vi "Image_set.vi"(8 "error in (no error)":errorcluster, 10 "Image":T1) -> (0 "error out":errorcluster)   [LabVIEW 2009, in "NetworkVarTarget.lvlib"]
uses:
  NetworkVarTarget.lvlib
  <vilib>/vision/Image Controls.llb/IMAQ Image.ctl
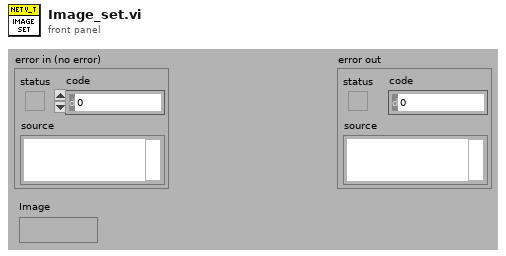
[diagram p1: front panel]
types:
  T1 = typedef "IMAQ Image.ctl" = refnum<image>
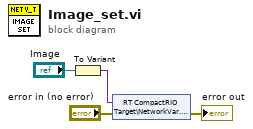
[diagram p0: block diagram]
diagram:
  n1 = To Variant(anything="Image") -> (Variant=w1:variant)
  n2 = shared-variable "RT CompactRIO Target\\NetworkVar.lvlib\\Image"(w1, error in="error in (no error)") -> (error out=→"error out":errorcluster)
